vi "RPC Method Manager Ping.vi"(8 "error in (no error)":errorcluster, 11 "OOP Server in":refnum<class "Manager.lvclass">) -> (0 "error out":errorcluster, 3 "OOP Server out":refnum<class "Manager.lvclass">)   [LabVIEW 2021, in "CIF_Manager_server.lvlib" / "Manager.lvclass"]
uses:
  Manager.lvclass
  Manager.lvclass/Manager.ctl
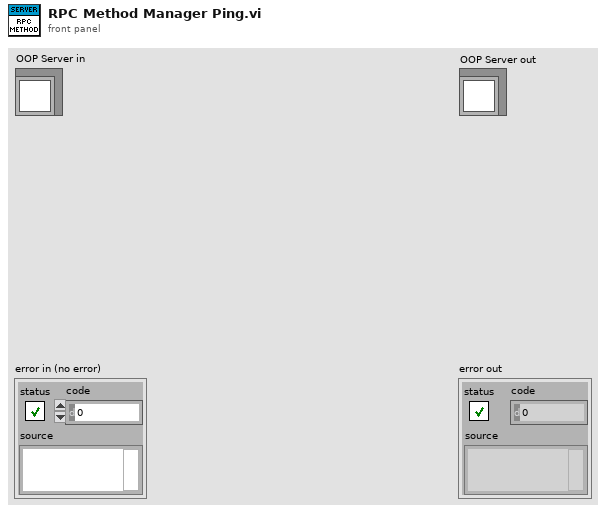
[diagram p1: front panel]
types:
  T1 = typedef "CIF_Manager_server.lvlib/Manager.lvclass/Server Internal UEs.ctl" = cluster{"Manager LoadPlugin Internal UE":refnum<user-event>, "Manager RegisterPlugin Internal UE":refnum<user-event>, "Manager UnregisterPlugin Internal UE":refnum<user-event>, "Manager QueryPluginTypes Internal UE":refnum<user-event>, "Manager AbortPlugin Internal UE":refnum<user-event>, "Manager UnloadAllPlugins Internal UE":refnum<user-event>, "Manager Destroy Internal UE":refnum<user-event>, "Manager Ping Internal UE":refnum<user-event>, "Manager QueryErrors Internal UE":refnum<user-event>, "Manager QueryConfig Internal UE":refnum<user-event>, "Manager QueryInfo Internal UE":refnum<user-event>, "Manager ResetErrorIndex Internal UE":refnum<user-event>, "Manager ResetConfigIndex Internal UE":refnum<user-event>, "Manager ResetInfoIndex Internal UE":refnum<user-event>, "Manager QueryPluginInfo Internal UE":refnum<user-event>, "Manager QueryPlugin Internal UE":refnum<user-event>}
  T2 = typedef "CIF_Manager_server.lvlib/Manager.lvclass/Server gRPC UEs.ctl" = cluster{"Manager LoadPlugin gRPC UE":refnum<user-event>, "Manager RegisterPlugin gRPC UE":refnum<user-event>, "Manager UnregisterPlugin gRPC UE":refnum<user-event>, "Manager QueryPluginTypes gRPC UE":refnum<user-event>, "Manager AbortPlugin gRPC UE":refnum<user-event>, "Manager UnloadAllPlugins gRPC UE":refnum<user-event>, "Manager Destroy gRPC UE":refnum<user-event>, "Manager Ping gRPC UE":refnum<user-event>, "Manager QueryErrors gRPC UE":refnum<user-event>, "Manager QueryConfig gRPC UE":refnum<user-event>, "Manager QueryInfo gRPC UE":refnum<user-event>, "Manager ResetErrorIndex gRPC UE":refnum<user-event>, "Manager ResetConfigIndex gRPC UE":refnum<user-event>, "Manager ResetInfoIndex gRPC UE":refnum<user-event>, "Manager QueryPluginInfo gRPC UE":refnum<user-event>, "Manager QueryPlugin gRPC UE":refnum<user-event>}
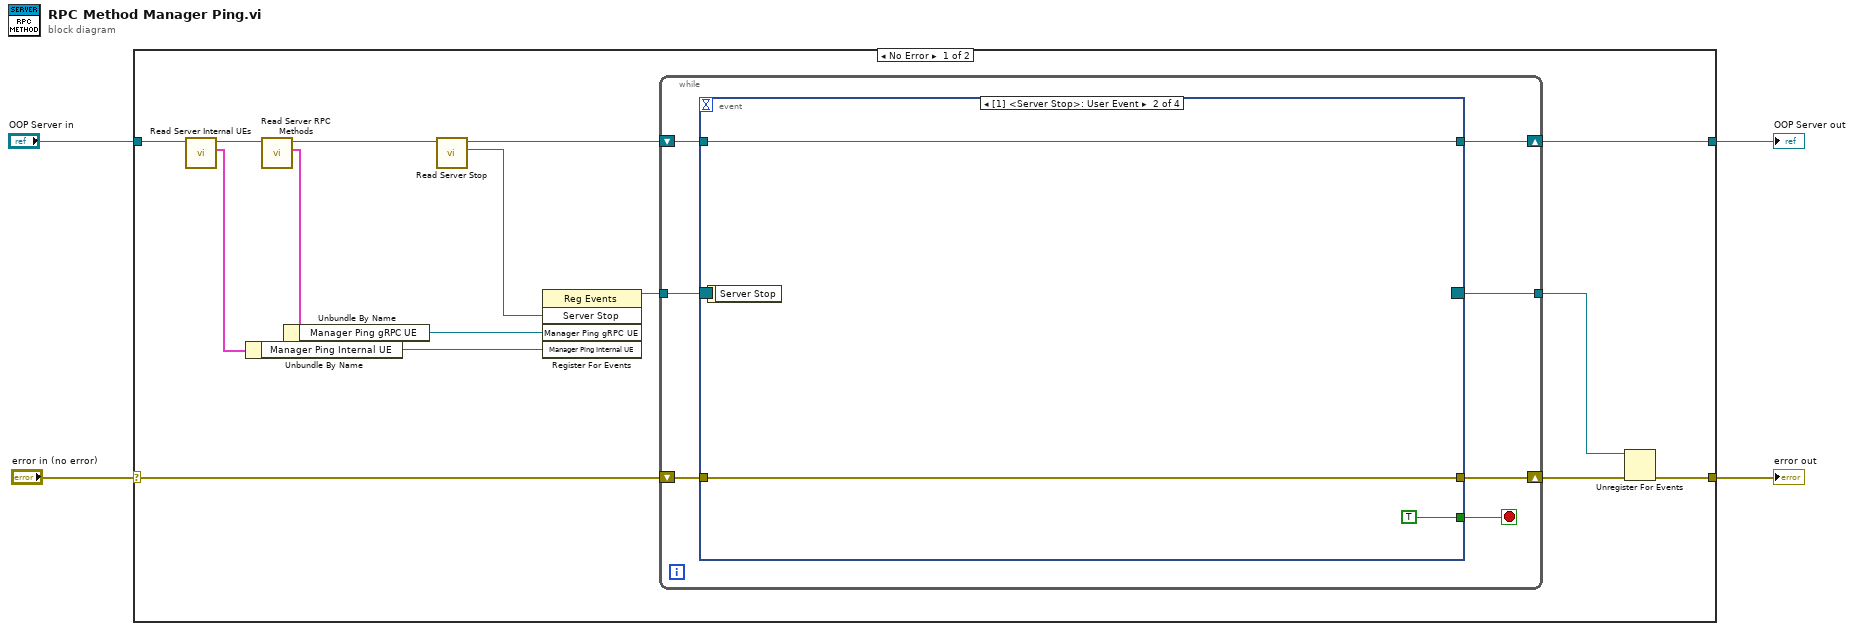
[diagram p0: block diagram]
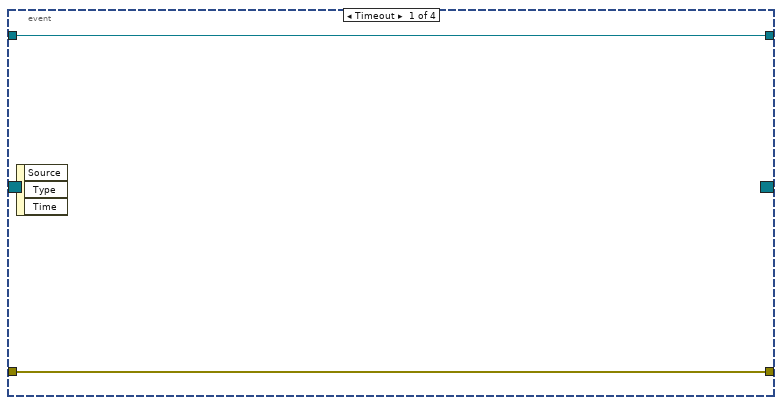
[diagram p2: hidden frame]
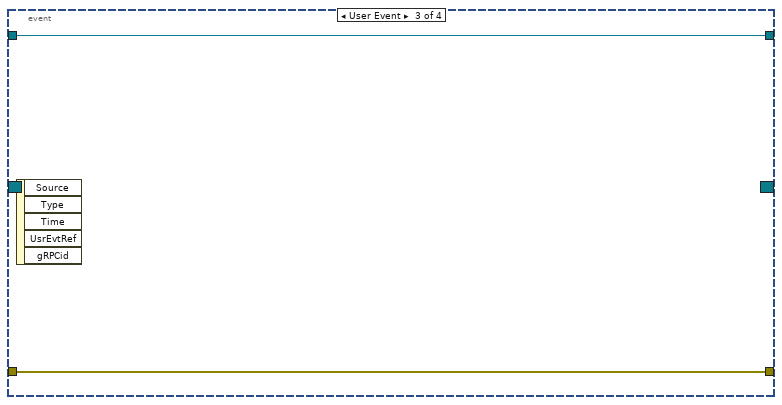
[diagram p3: hidden frame]
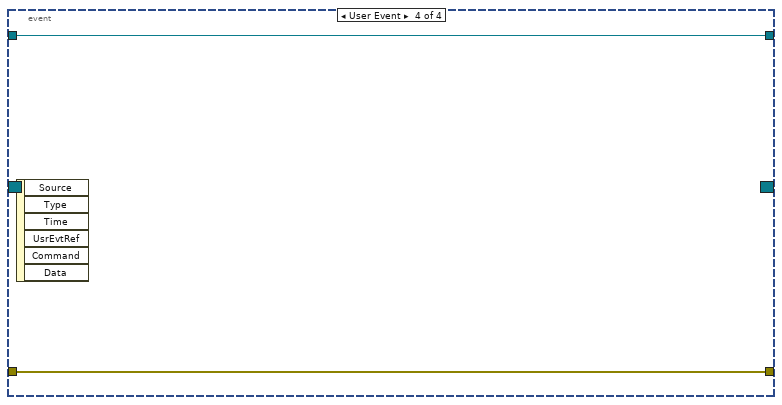
[diagram p4: hidden frame]
diagram:
  n1 = case shown="No Error" "error in (no error)" {
    selector: "error in (no error)" -> [w15 w37]
    tunnel: [w13 w37] -> w3
    tunnel: "OOP Server in" -> [w17 w36]
    tunnel: [w5 w36] -> w1
    frame No Error {
      n2 = call "Read Server Internal UEs.vi"("SignalGeneratorService in"=w17) -> ("Server Internal UEs"=w9:T1, "SignalGeneratorService out"=w16:refnum<class "Manager.lvclass">)  [unwired: 8 in, 1 out]
      n3 = Unbundle By Name ("Unbundle Internal UE")(w9) -> ("Manager Ping Internal UE"=w8:refnum<user-event>)
      n4 = call "Read Server RPC Methods.vi"("SignalGeneratorService in"=w16) -> ("Server RPC Methods"=w11:T2, "SignalGeneratorService out"=w6:refnum<class "Manager.lvclass">)  [unwired: 8 in, 1 out]
      n5 = Unbundle By Name ("Unbundle gRPC UE")(w11) -> ("Manager Ping gRPC UE"=w10:refnum<user-event>)
      n6 = call-dynamic "Read Server Stop.vi"("iService in"=w6) -> ("Server Stop"=w19:refnum<user-event>, "iService out"=w7:refnum<class "Manager.lvclass">)  [unwired: 8 in, 1 out]
      n7 = register-events(w19, w10, w8) -> (reference out=w18:refnum<event-registration>)  [unwired: 2 in, 1 out]
      n8 = while {
        tunnel: w18 -> [w26]
        tunnel: [w22] -> w12
        shift-right: [w23] -> w14
        shift-left: w15 -> [w24]
        shift-right: [w20] -> w5
        shift-left: w7 -> [w21]
        stop <- w25 stop-if-true
        n9 = event "RPC Method Event Structure" shown="[1] <Server Stop>: User Event" {
          selector: w26 -> [_ _ _ _]
          dyn-events: [_ _ _ _] -> w22
          timeout: _ -> [_ _ _ _]
          tunnel: [_ TRUE _ _] -> w25
          tunnel: w24 -> [w28 w30 w33 w35]
          tunnel: [w28 w30 w33 w35] -> w23
          tunnel: w21 -> [w27 w29 w32 w34]
          tunnel: [w27 w29 w32 w34] -> w20
          event Timeout {
            n10 = event-data() -> ()  [unwired: 1 in, 3 out]
          }
          event User Event {
            n11 = event-data() -> ()  [unwired: 1 in, 1 out]
          }
          event User Event {
            n12 = event-data() -> ()  [unwired: 1 in, 5 out]
          }
          event User Event {
            n13 = event-data() -> ()  [unwired: 1 in, 6 out]
          }
        }
      }
      n14 = Unregister For Events(event registration refnum=w12, error in=w14) -> (error out=w13:errorcluster)
    }
    frame Error {
    }
  }
  "error out" <- w3
  "OOP Server out" <- w1
